vi "Read Boolean.vi"(8 "error in (no error)":errorcluster, 10 "Label":string, 11 "FlexWorktable in":refnum<class "FlexWorktable.lvclass">) -> (0 "error out":errorcluster, 2 "Boolean":bool=TRUE, 3 "FlexWorktable out":refnum<class "FlexWorktable.lvclass">)   [LabVIEW 2017, in "FlexWorktable.lvclass"]
uses:
  FlexWorktable.lvclass
  FlexWorktable.lvclass/FlexWorktable.ctl
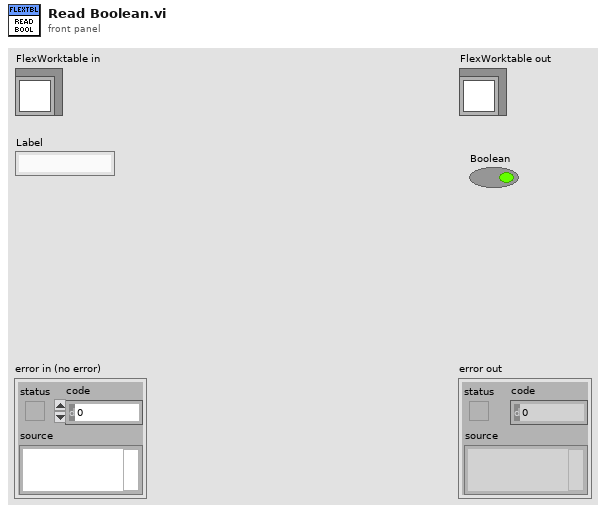
[diagram p1: front panel]
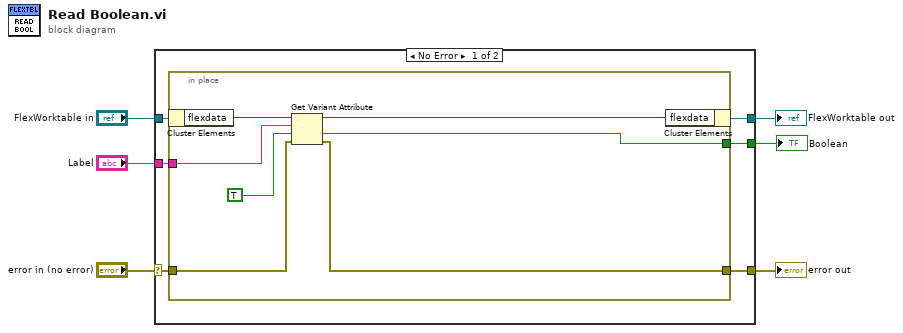
[diagram p0: block diagram]
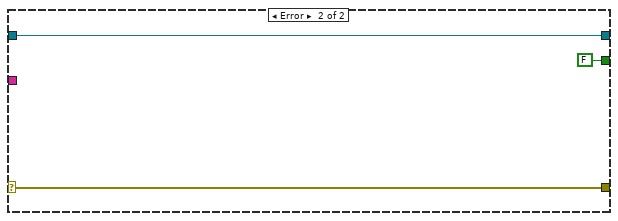
[diagram p2: hidden frame]
diagram:
  n1 = case shown="No Error" "error in (no error)" {
    selector: "error in (no error)" -> [w11 w22]
    tunnel: [w9 w22] -> w5
    tunnel: [w8 w21] -> w3
    tunnel: "FlexWorktable in" -> [w12 w21]
    tunnel: "Label" -> [w10 _]
    tunnel: [w7 FALSE] -> w1
    frame No Error {
      n2 = in-place {
        in-place-border: w11 -> [w15]
        in-place-border: w10 -> [w18]
        in-place-border: [w16] -> w9
        in-place-border: [w13] -> w7
        n3 = in-place-cluster #1(w12) -> ("flexdata"=w19:variant)
        n4 = Get Variant Attribute(Variant=w19, name=w18, default value (empty Variant)=TRUE, error in=w15) -> (duplicate Variant=w17:variant, value=w13:bool, error out=w16:errorcluster)  [unwired: 1 out]
        n5 = in-place-cluster #1("flexdata"=w17) -> (w8:refnum<class "FlexWorktable.lvclass">)
      }
    }
    frame Error {
    }
  }
  "error out" <- w5
  "FlexWorktable out" <- w3
  "Boolean" <- w1
